vi "Lab Panel V6.00.vi"() -> ()   [LabVIEW 2017]
uses:
  sub vi/SelectLAB0X-N.ctl
  sub vi/SIG LAB0X-N.ctl
  sub vi/Set LAB0X-N.ctl
  <vilib>/Platform/TimedLoop/XDataNode/timing_clust.ctl
  <vilib>/Platform/TimedLoop/XDataNode/nitl_modes.ctl
  <vilib>/Platform/TimedLoop/XDataNode/wakeup.ctl
  Global 1.vi
  Global display 4.vi
  Global display 3.vi
  Global display 1.vi
  Global display 2.vi
  <vilib>/platform/TimedLoop/XDataNode/XDataNode.xnode
  <vilib>/Platform/TimedLoop/XDataNode/XDNodeRunTimeDep.lvlib
  sub vi/Web Imge control.ctl
panel:
  out "Loop Time":u32
  out "Process AIs":bool
  in  "path to JPEG file":path=path "C:/Users/Mike/Documents/Crabtree/Crabtree/Hardware/crabtree"
  out "Simulate IND":bool
  out "network error":bool
  out "TEMP":bool
  out "AI":bool
  out "Amb Temp":dbl format="%#.0f"
  out "Temp Up":dbl
  in  "stop all":bool
  in  "ADMIN":bool
  in  "Tab Control 2":T1(tab)
  out "SIG LAB05-2":T2 {"PF" format="%.2f"; "AMPS" format="%.1f"}
  out "SIG LAB05-1":T2 {"PF" format="%.2f"; "AMPS" format="%.1f"}
  out "SIG LAB04-2":T2 {"PF" format="%.2f"; "AMPS" format="%.1f"}
  out "SIG LAB04-1":T2 {"PF" format="%.2f"; "AMPS" format="%.1f"}
  out "SIG LAB03-2":T2 {"PF" format="%.2f"; "AMPS" format="%.1f"}
  out "SIG LAB03-1":T2 {"PF" format="%.2f"; "AMPS" format="%.1f"}
  out "SIG LAB02-2":T2 {"PF" format="%.2f"; "AMPS" format="%.1f"}
  in  "RUN LAB01-1":bool
  in  "O/I  LAB05-1":bool
  in  "O/I  LAB05-2":bool
  in  "O/I  LAB04-1":bool
  in  "O/I  LAB04-2":bool
  in  "O/I  LAB02-1":bool
  in  "O/I  LAB02-2":bool
  in  "O/I  LAB01-2":bool
  in  "O/I  LAB01-1":bool
  in  "O/I  LAB03-1":bool
  in  "RUN LAB05-2":bool
  in  "RUN LAB05-1":bool
  in  "RUN LAB04-2":bool
  in  "RUN LAB04-1":bool
  in  "RUN LAB03-2":bool
  in  "RUN LAB03-1":bool
  in  "RUN LAB02-2":bool
  in  "RUN LAB02-1":bool
  in  "RUN LAB01-2":bool
  in  "SELECT LAB05-2":T3
  in  "SELECT LAB05-1":T3
  in  "SELECT LAB04-2":T3
  in  "SELECT LAB04-1":T3
  in  "SELECT LAB03-2":T3
  in  "SELECT LAB03-1":T3
  in  "SELECT LAB02-2":T3
  in  "SELECT LAB02-1":T3
  in  "SELECT LAB01-2":T3
  in  "SELECT LAB01-1":T3
  in  "O/I  LAB03-2":bool
  out "SIG LAB01-1":T2 {"PF" format="%.2f"; "AMPS" format="%.1f"}
  out "SIG LAB01-2":T2 {"PF" format="%.2f"; "AMPS" format="%.1f"}
  out "SIG LAB02-1":T2 {"PF" format="%.2f"; "AMPS" format="%.1f"}
  out "DISP LAB05-2":T4 {"MINS" format="%.2g"}
  out "DISP LAB05-1":T4 {"MINS" format="%.2g"}
  out "DISP LAB04-2":T4 {"MINS" format="%.2g"}
  out "DISP LAB04-1":T4 {"MINS" format="%.2g"}
  out "DISP LAB03-2":T4 {"MINS" format="%.2g"}
  out "DISP LAB03-1":T4 {"MINS" format="%.2g"}
  in  "SET LAB05-2":T5={"NAME"="", "DESCRIPTION"="", "CYCLES"=5.0, "T-RISE mins"=0.0, "T-RISE deg C"=0.0} {"CYCLES" min=5.0 step=1.0}
  in  "SET LAB05-1":T5={"NAME"="", "DESCRIPTION"="", "CYCLES"=5.0, "T-RISE mins"=0.0, "T-RISE deg C"=0.0} {"CYCLES" min=5.0 step=1.0}
  in  "SET LAB04-2":T5={"NAME"="", "DESCRIPTION"="", "CYCLES"=5.0, "T-RISE mins"=0.0, "T-RISE deg C"=0.0} {"CYCLES" min=5.0 step=1.0}
  in  "SET LAB04-1":T5={"NAME"="", "DESCRIPTION"="", "CYCLES"=5.0, "T-RISE mins"=0.0, "T-RISE deg C"=0.0} {"CYCLES" min=5.0 step=1.0}
  in  "SET LAB03-2":T5={"NAME"="", "DESCRIPTION"="", "CYCLES"=5.0, "T-RISE mins"=0.0, "T-RISE deg C"=0.0} {"CYCLES" min=5.0 step=1.0}
  in  "SET LAB03-1":T5={"NAME"="", "DESCRIPTION"="", "CYCLES"=5.0, "T-RISE mins"=0.0, "T-RISE deg C"=0.0} {"CYCLES" min=5.0 step=1.0}
  out "DISP LAB02-2":T4 {"MINS" format="%.2g"}
  out "DISP LAB02-1":T4 {"MINS" format="%.2g"}
  in  "SET LAB02-2":T5={"NAME"="", "DESCRIPTION"="", "CYCLES"=5.0, "T-RISE mins"=0.0, "T-RISE deg C"=0.0} {"CYCLES" min=5.0 step=1.0}
  in  "SET LAB02-1":T5={"NAME"="", "DESCRIPTION"="", "CYCLES"=5.0, "T-RISE mins"=0.0, "T-RISE deg C"=0.0} {"CYCLES" min=5.0 step=1.0}
  out "RESULT LAB05-2":bool
  out "RESULT LAB05-1":bool
  out "RESULT LAB04-2":bool
  out "RESULT LAB04-1":bool
  out "RESULT LAB03-2":bool
  out "RESULT LAB03-1":bool
  out "RESULT LAB02-2":bool
  out "RESULT LAB02-1":bool
  out "RESULT LAB01-2":bool
  out "RESULT LAB01-1":bool
  in  "SET LAB01-1":T6={"NAME"="", "DESCRIPTION"="", "CYCLES"=5.0, "T-RISE mins"=0.0, "T-RISE deg C"=0.0} {"CYCLES" min=5.0 step=1.0}
  in  "SET LAB01-2":T5={"NAME"="", "DESCRIPTION"="", "CYCLES"=5.0, "T-RISE mins"=0.0, "T-RISE deg C"=0.0} {"CYCLES" min=5.0 step=1.0}
  out "DISP LAB01-1":T4 {"MINS" format="%.2g"}
  out "DISP LAB01-2":T4 {"MINS" format="%.2f"}
  out "TEMP RISE LAB05-2":cluster{"TL":dbl, "TN":dbl}
  out "TEMP RISE LAB05-1":cluster{"TL":dbl, "TN":dbl}
  out "TEMP RISE LAB04-2":cluster{"TL":dbl, "TN":dbl}
  out "TEMP RISE LAB04-1":cluster{"TL":dbl, "TN":dbl}
  out "TEMP RISE LAB03-2":cluster{"TL":dbl, "TN":dbl}
  out "TEMP RISE LAB03-1":cluster{"TL":dbl, "TN":dbl}
  out "TEMP RISE LAB02-2":cluster{"TL":dbl, "TN":dbl}
  out "TEMP RISE LAB02-1":cluster{"TL":dbl, "TN":dbl}
  out "TEMP RISE LAB01-2":cluster{"TL":dbl, "TN":dbl}
  out "TEMP RISE LAB01-1":cluster{"TL":dbl, "TN":dbl}
  out "JIG LAB05-2":bool
  out "JIG LAB05-1":bool
  out "JIG LAB04-2":bool
  out "JIG LAB04-1":bool
  out "JIG LAB03-2":bool
  out "JIG LAB03-1":bool
  out "JIG LAB02-2":bool
  out "JIG LAB02-1":bool
  out "JIG LAB01-2":bool
  out "JIG LAB01-1":bool
  out "TEMP START LAB01-1":cluster{"TL":dbl, "TN":dbl}
  out "TEMP START LAB02-1":cluster{"TL":dbl, "TN":dbl}
  out "TEMP START LAB03-1":cluster{"TL":dbl, "TN":dbl}
  out "TEMP START LAB04-1":cluster{"TL":dbl, "TN":dbl}
  out "TEMP START LAB01-2":cluster{"TL":dbl, "TN":dbl}
  out "TEMP START LAB02-2":cluster{"TL":dbl, "TN":dbl}
  out "TEMP START LAB03-2":cluster{"TL":dbl, "TN":dbl}
  out "TEMP START LAB04-2":cluster{"TL":dbl, "TN":dbl}
  out "TEMP START LAB05-2":cluster{"TL":dbl, "TN":dbl}
  out "TEMP START LAB05-1":cluster{"TL":dbl, "TN":dbl}
  out "LOG LAB05-2":string
  out "LOG LAB04-2":string
  out "LOG LAB03-2":string
  out "LOG LAB02-2":string
  out "LOG LAB01-2":string
  out "LOG LAB05-1":string
  out "LOG LAB04-1":string
  out "LOG LAB03-1":string
  out "LOG LAB02-1":string
  out "LOG LAB01-1":string
  in  "Tab charts":T7(tab)
  out "LAB01 VOLTS":dynamicdata(graph)
  out "LAB01 AMPS":dynamicdata(graph)
  out "LAB01 deg C":dynamicdata(graph)
  out "LAB02 VOLTS":dynamicdata(graph)
  out "LAB02 AMPS":dynamicdata(graph)
  out "LAB02 deg C":dynamicdata(graph)
  out "LAB03 VOLTS":dynamicdata(graph)
  out "LAB03 AMPS":dynamicdata(graph)
  out "LAB03 deg C":dynamicdata(graph)
  out "LAB04 VOLTS":dynamicdata(graph)
  out "LAB04 AMPS":dynamicdata(graph)
  out "LAB04 deg C":dynamicdata(graph)
  out "LAB05 VOLTS":dynamicdata(graph)
  out "LAB05 AMPS":dynamicdata(graph)
  out "LAB05 deg C":dynamicdata(graph)
  out "Reset Error":bool
  out "Er USB#2":dbl
  out "Er USB#1":dbl
  out "Er USB#0":dbl
  out "Resets Done":dbl
  out "Error USB #2":bool
  out "Error USB #1":bool
  out "Error USB #0":bool
  in  "MAIL SETTINGS":T8
  out "MAIL REPORT":string
  in  "TO (string):":string
  in  "Send Mail Now":bool
  in  "Auto Mail Send":bool
  in  "Network Directory":path
  in  "JIG ON TIME (S)":dbl=1.0 min=1.0 max=10.0 step=0.5 format="%.1g"
  in  "JIG OFF TIME (S)":dbl=2.0 min=2.0 max=10.0 step=0.5 format="%.1g"
  in  "Reset Measuring":bool
  out "path":path
  out "physical channels 0":string="DemoDevice,BID#0/ai0:1" caption="property value"
  out "physical channels 1":string="DemoDevice,BID#0/ai0:1" caption="property value"
  out "physical channels 2":string="DemoDevice,BID#0/ai0:1" caption="property value"
  in  "Min I":dbl=1.0
  in  "Min V":dbl=10.0
  out "JIG RELAY CYCLES":T9
  out "ON L05-2":cluster{"amps":dbl, "volts":dbl, "pf":dbl}
  out "ON L05-1":cluster{"amps":dbl, "volts":dbl, "pf":dbl}
  out "FAIL LAB05-2":cluster{"LO":dbl, "HI":dbl}
  out "FAIL LAB05-1":cluster{"LO":dbl, "HI":dbl}
  out "FAIL LAB04-2":cluster{"LO":dbl, "HI":dbl}
  out "FAIL LAB04-1":cluster{"LO":dbl, "HI":dbl}
  out "FAIL LAB03-2":cluster{"LO":dbl, "HI":dbl}
  out "FAIL LAB03-1":cluster{"LO":dbl, "HI":dbl}
  out "FAIL LAB02-2":cluster{"LO":dbl, "HI":dbl}
  out "FAIL LAB02-1":cluster{"LO":dbl, "HI":dbl}
  out "FAIL LAB01-2":cluster{"LO":dbl, "HI":dbl}
  out "FAIL LAB01-1":cluster{"LO":dbl, "HI":dbl}
  out "ON L01-1":cluster{"amps":dbl, "volts":dbl, "pf":dbl}
  out "ON L01-2":cluster{"amps":dbl, "volts":dbl, "pf":dbl}
  out "ON L02-1":cluster{"amps":dbl, "volts":dbl, "pf":dbl}
  out "ON L02-2":cluster{"amps":dbl, "volts":dbl, "pf":dbl}
  out "ON L03-1":cluster{"amps":dbl, "volts":dbl, "pf":dbl}
  out "ON L03-2":cluster{"amps":dbl, "volts":dbl, "pf":dbl}
  out "ON L04-1":cluster{"amps":dbl, "volts":dbl, "pf":dbl}
  out "ON L04-2":cluster{"amps":dbl, "volts":dbl, "pf":dbl}
  in  "Open Com Port":bool
  out "LA05-2 (TN)":bool
  out "LA05-2 (TL)":bool
  out "LA05-1 (TN)":bool
  out "LA05-1 (TL)":bool
  out "LA04-2 (TN)":bool
  out "LA04-2 (TL)":bool
  out "LA04-1 (TN)":bool
  out "LA04-1 (TL)":bool
  out "LA03-2 (TN)":bool
  out "LA03-2 (TL)":bool
  out "LA03-1 (TN)":bool
  out "LA03-1 (TL)":bool
  out "LA02-2 (TN)":bool
  out "LA02-2 (TL)":bool
  out "LA02-1 (TN)":bool
  out "LA02-1 (TL)":bool
  out "LA01-2 (TN)":bool
  out "LA01-2 (TL)":bool
  out "LA01-1 (TN)":bool
  out "LA01-1 (TL)":bool
  out "TEMP LA05":T10
  out "TEMP LA04":T10
  out "TEMP LA03":T10
  out "TEMP LA02":T10
  out "TEMP LA01":T10
  out "Ref deg C":dbl format="%#.0f"
  out "Temp read loop":dbl
  out "Com Port Status":bool
  out "Com setup loops":i32
  out "VISA Com out":refnum<visa-resource-name>
  in  "Select COM port":refnum<visa-resource-name>="COM6"
  in  "Read Temp":bool
  out "Error Temp":bool
  out "Fault Counters":u64[](array[numeric])
  out "TempErrors":bool[](array[boolean])
  in  "Temp Simulate":bool
  out "AI Task":bool
  out "AI Task2":u32
  out "AI Task1":u32
  out "AI Task0":u64
  out "Total USB resets":dbl
  in  "Auto Reset":bool
  in  "Mail Test File To:":string
  in  "Mail Test Fail":bool
  out "graph flag":bool
  in  "Temp Test Cal":dbl
  in  "Amps Fail level":dbl
  in  "Fail Loops":dbl
  out "Save JC":bool
  in  "DAQ Simulate":bool
  in  "Temp Value":dbl
  in  "Temp Delay Lps":dbl
  in  "SAMPLES":dbl
  in  "RATE (Hz)":dbl
  in  "JIG TEST":T11
  in  "C drive data root dir":path
  out "run lab05-2":bool
  out "run lab05-1":bool
  out "run lab04-2":bool
  out "run lab04-1":bool
  out "run lab03-2":bool
  out "run lab03-1":bool
  out "run lab02-2":bool
  out "run lab02-1":bool
  out "run lab01-2":bool
  out "run lab01-1":bool
  in  "Tab Control":T12(tab)
  out "LAB01-2 (GRAPH)":dynamicdata(graph)
  out "LAB01-1 (GRAPH)":dynamicdata(graph)
  out "LAB02-2 (GRAPH)":dynamicdata(graph)
  out "LAB02-1 (GRAPH)":dynamicdata(graph)
  out "LAB03-2 (GRAPH)":dynamicdata(graph)
  out "LAB03-1 (GRAPH)":dynamicdata(graph)
  out "LAB04-2 (GRAPH)":dynamicdata(graph)
  out "LAB04-1 (GRAPH)":dynamicdata(graph)
  out "LAB05-2 (GRAPH)":dynamicdata(graph)
  out "LAB05-1 (GRAPH)":dynamicdata(graph)
  out "Any Test Running":bool
  out "Read Time":dbl
  out "LAB05 TEMP":T13
  out "LAB04 TEMP":T13
  out "LAB02 TEMP":T13
  out "LAB01 TEMP":T13
  out "LAB03 TEMP":T13
  out "LAB05-TP":bool
  out "LAB04-TP":bool
  out "LAB03-TP":bool
  out "LAB02-TP":bool
  out "LAB01-TP":bool
  out "Analog error":bool
  out "USB OUT 0":bool[](array[boolean])
  out "USB OUT 1":bool[](array[boolean])
  out "USB OUT 2":bool[](array[boolean])
  in  "Ambient Volts":dbl format="%.2f"
  in  "PF":dbl min=0.0 max=1.0 step=0.1 format="%#.1f"
  in  "VOLTS":dbl
  in  "OFF amps":dbl min=0.0 max=100.0 step=0.1 format="%#.1f"
  in  "ON amps":dbl
  in  "LAB deg C":T14
  out "AI data 0":waveform(dbl)[](array[waveform])
  out "AI data 1":waveform(dbl)[](array[waveform])
  out "AI data 2":waveform(dbl)[](array[waveform])
  out "AI Error":errorcluster[](array[cluster])
  out "AI loop time":dbl format="%.6g"
  out "loops":dbl
  out "on loops":dbl format="%#.0f"
  out "off loops":dbl format="%#.0f"
  out "jig cycle":dbl
  out "TDMS LAB01-1":refnum<k34>
  out "data file error":errorcluster
  out "TDMS LAB02-1":refnum<k34>
  out "TDMS LAB01-2":refnum<k34>
  out "TDMS LAB02-2":refnum<k34>
  out "TDMS LAB03-1":refnum<k34>
  out "TDMS LAB03-2":refnum<k34>
  out "TDMS LAB04-1":refnum<k34>
  out "TDMS LAB04-2":refnum<k34>
  out "TDMS LAB05-1":refnum<k34>
  out "TDMS LAB05-2":refnum<k34>
  out "mail control":string
  out "File Time Stamp":timestamp
  in  "stop":bool
  out "deg C (volts)":dbl
  out "Application Directory":path
  out "ACQ Init TIme":u32
  out "ACQ Time":u32
  out "Web Server:Root Directory Path":path
  out "Analog Fault Counts":i32[](array[numeric])
  out "TEMP REF cal":dbl
  out "CAL LAB01":T15 {"2 (TN) cal" min=0.0 step=0.01 format="%.2f"; "2 (TL) cal" min=0.0 step=0.01 format="%.2f"; "2 (PF) cal" min=0.0 step=0.01 format="%.2f"; "2 (V) cal" min=0.0 step=0.01 format="%.2f"; "2 (A) cal" min=0.0 step=0.01 format="%.2f"; "1 (TN) cal" min=0.0 step=0.01 format="%.2f"; "1 (TL) cal" min=0.0 step=0.01 format="%.2f"; "1 (PF) cal" min=0.0 step=0.01 format="%.2f"; "1 (V) cal" min=0.0 step=0.01 format="%.2f"; "1  (A) cal" min=0.0 step=0.01 format="%.2f"}
  out "CAL LAB03":T15 {"2 (TN) cal" min=0.0 step=0.01 format="%.2f"; "2 (TL) cal" min=0.0 step=0.01 format="%.2f"; "2 (PF) cal" min=0.0 step=0.01 format="%.2f"; "2 (V) cal" min=0.0 step=0.01 format="%.2f"; "2 (A) cal" min=0.0 step=0.01 format="%.2f"; "1 (TN) cal" min=0.0 step=0.01 format="%.2f"; "1 (TL) cal" min=0.0 step=0.01 format="%.2f"; "1 (PF) cal" min=0.0 step=0.01 format="%.2f"; "1 (V) cal" min=0.0 step=0.01 format="%.2f"; "1  (A) cal" min=0.0 step=0.01 format="%.2f"}
  out "CAL LAB02":T16 {"2 (TN) cal" min=0.0 step=0.01 format="%.2f"; "2 (TL) cal" min=0.0 step=0.01 format="%.2f"; "2 (PF) cal" min=0.0 step=0.01 format="%.2f"; "2 (V) cal" min=0.0 step=0.01 format="%.2f"; "2 (A) cal" min=0.0 step=0.01 format="%.2f"; "1 (TN) cal" min=0.0 step=0.01 format="%.2f"; "1 (TL) cal" min=0.0 step=0.01 format="%.2f"; "1 (PF) cal" min=0.0 step=0.01 format="%.2f"; "1 (V) cal" min=0.0 step=0.01 format="%.2f"; "1 (A) cal" min=0.0 step=0.01 format="%.2f"}
  out "CAL LAB05":T15 {"2 (TN) cal" min=0.0 step=0.01 format="%.2f"; "2 (TL) cal" min=0.0 step=0.01 format="%.2f"; "2 (PF) cal" min=0.0 step=0.01 format="%.2f"; "2 (V) cal" min=0.0 step=0.01 format="%.2f"; "2 (A) cal" min=0.0 step=0.01 format="%.2f"; "1 (TN) cal" min=0.0 step=0.01 format="%.2f"; "1 (TL) cal" min=0.0 step=0.01 format="%.2f"; "1 (PF) cal" min=0.0 step=0.01 format="%.2f"; "1 (V) cal" min=0.0 step=0.01 format="%.2f"; "1  (A) cal" min=0.0 step=0.01 format="%.2f"}
  out "CAL LAB04":T15 {"2 (TN) cal" min=0.0 step=0.01 format="%.2f"; "2 (TL) cal" min=0.0 step=0.01 format="%.2f"; "2 (PF) cal" min=0.0 step=0.01 format="%.2f"; "2 (V) cal" min=0.0 step=0.01 format="%.2f"; "2 (A) cal" min=0.0 step=0.01 format="%.2f"; "1 (TN) cal" min=0.0 step=0.01 format="%.2f"; "1 (TL) cal" min=0.0 step=0.01 format="%.2f"; "1 (PF) cal" min=0.0 step=0.01 format="%.2f"; "1 (V) cal" min=0.0 step=0.01 format="%.2f"; "1  (A) cal" min=0.0 step=0.01 format="%.2f"}
  out "cal file error out":errorcluster
  in  "SET (cal)":bool
  out "AI Data 0":waveform(dbl)[](graph)
  out "AI Data 1":waveform(dbl)[](graph)
  out "AI Data 2":waveform(dbl)[](graph)
  # "v6.28"
  # "LAB01"
  # "LAB02"
  # "LAB03"
  # "LAB04"
  # "LAB05"
  # "LAB01"
  # "LAB02"
  # "LAB03"
  # "LAB04"
  # "LAB05"
  # "PANEL ID / DATE / TIME / NAME / DESCRIPTION / CYCLES / TEST TIME / STATUS"
  # "PANEL ID / DATE / TIME / NAME / DESCRIPTION / CYCLES / TEST TIME / STATUS"
  # "http://This IP:8000/Lab_Panel"
  # "(Enter recipients address seperated by comma)"
  # "JIG SET"
  # "Temperature circuits \ndetected at start up."
  # "PANEL CONTROL TO BE ON"
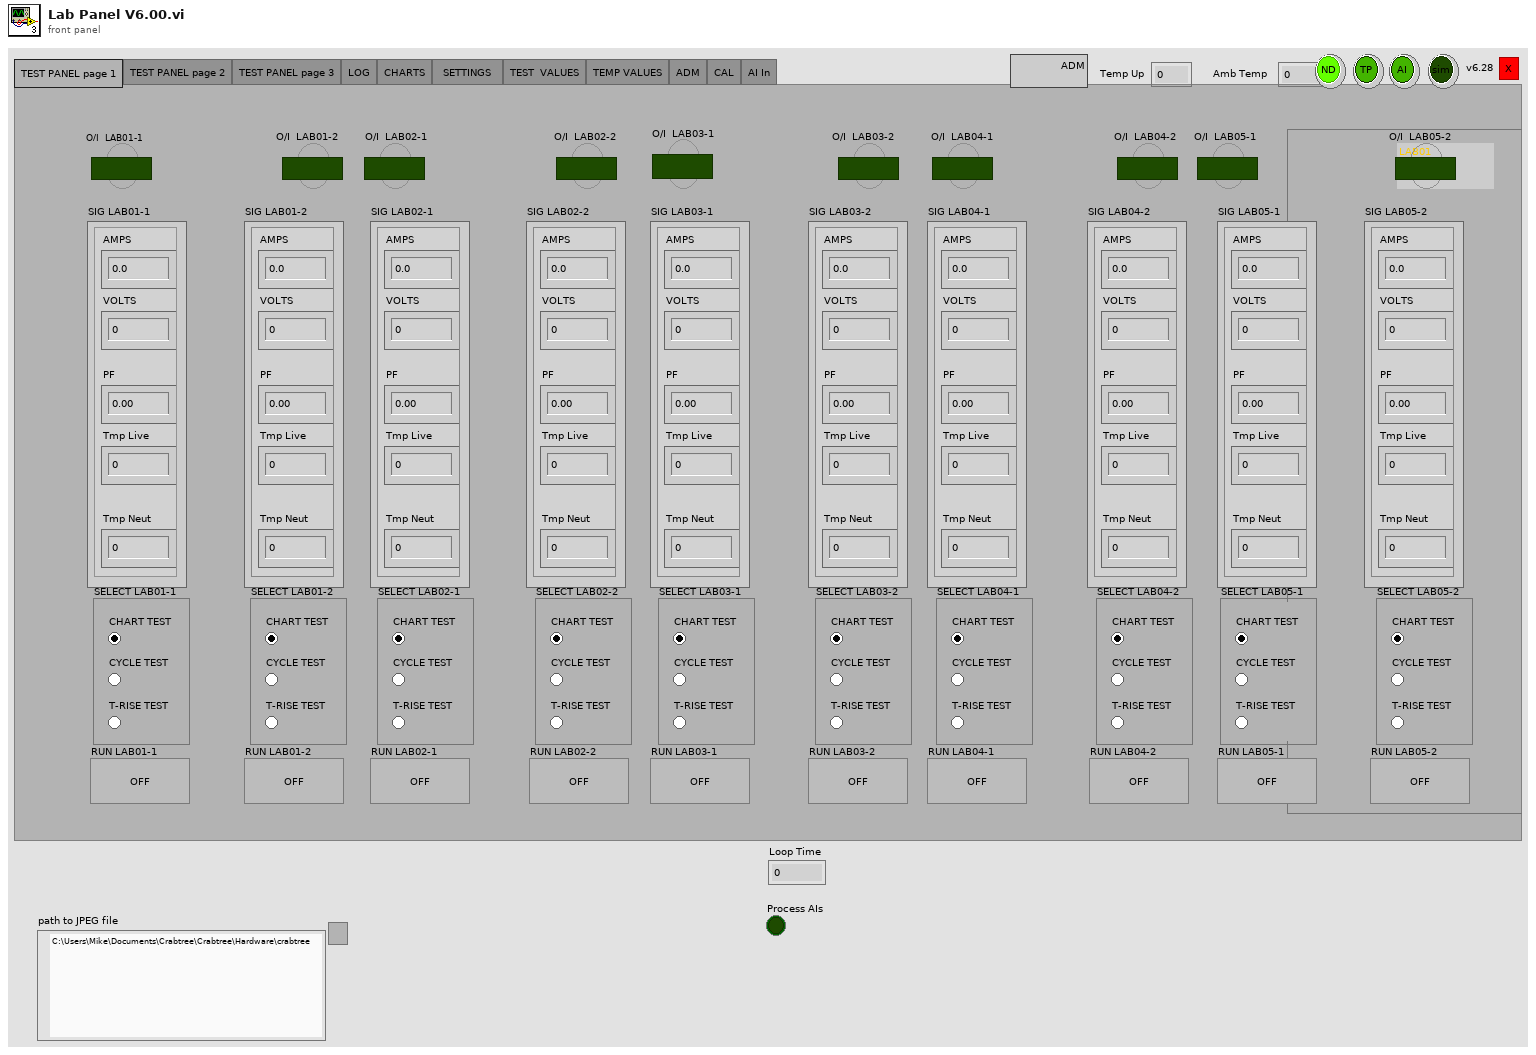
[diagram p1: front panel]
types:
  T1 = enum32{"TEST PANEL page 1", "TEST PANEL page 2", "TEST PANEL page 3", "LOG", "CHARTS", "SETTINGS   ", "TEST  VALUES", "TEMP VALUES", "ADM", "CAL", "AI In"}
  T2 = typedef "SIG LAB0X-N.ctl" = cluster{"AMPS":dbl, "VOLTS":dbl, "PF":dbl, "Tmp Live":dbl, "Tmp Neut":dbl}
  T3 = typedef "SelectLAB0X-N.ctl" = enum32{"CHART TEST", "CYCLE TEST", "T-RISE TEST"}
  T4 = cluster{"CYCLE":dbl, "MINS":dbl, "STATUS":string}
  T5 = cluster{"NAME":string, "DESCRIPTION":string, "CYCLES":dbl, "T-RISE mins":dbl, "T-RISE deg C":dbl}
  T6 = typedef "Set LAB0X-N.ctl" = cluster{"NAME":string, "DESCRIPTION":string, "CYCLES":dbl, "T-RISE mins":dbl, "T-RISE deg C":dbl}
  T7 = enum32{"LAB01", "LAB02", "LAB03", "LAB04", "LAB05"}
  T8 = cluster{"OUT SERVER ADDRESS":string, "FROM ACCOUNT":string, "USER NAME":string, "PASSWORD":string, "TEST MAIL":bool, "TEST MAIL STATUS":string, "mail error":errorcluster}
  T9 = cluster{"LAB01-1":dbl, "LAB01-2":dbl, "LAB02-1":dbl, "LAB02-2":dbl, "LAB03-1":dbl, "LAB03-2":dbl, "LAB04-1":dbl, "LAB04-2":dbl, "LAB05-1":dbl, "LAB05-2":dbl}
  T10 = cluster{"TL-1":dbl, "TN-1":dbl, "TL-2":dbl, "TN-2":dbl, "TL -1COUNT":dbl, "TN-1 COUNT":dbl, "TL-2 COUNT":dbl, "TN-2 COUNT":dbl}
  T11 = cluster{" LAB01-1":bool, " LAB01-2":bool, "LAB02-1":bool, " LAB02-2":bool, "LAB03-1":bool, "LAB03-2":bool, "LAB04-1":bool, "LAB04-2":bool, "LAB05-1":bool, "LAB05-2":bool}
  T12 = enum32{"LAB01", "LAB02", "LAB03", "LAB04", "LAB05", "TEMPERATURE", "GENERAL INFO", "Simulate", "AI Data Out"}
  T13 = cluster{"T1 Live":dbl, "T1 Neut":dbl, "T2 Live":dbl, "T2 Neut":dbl, "ID":dbl, "ER":dbl}
  T14 = cluster{"1 TL":dbl, "1 TN":dbl, "2 TL":dbl, "2 TN":dbl, "ID":dbl, "ER":dbl}
  T15 = cluster{"1  (A) cal":dbl, "1 (V) cal":dbl, "1 (PF) cal":dbl, "1 (TL) cal":dbl, "1 (TN) cal":dbl, "2 (A) cal":dbl, "2 (V) cal":dbl, "2 (PF) cal":dbl, "2 (TL) cal":dbl, "2 (TN) cal":dbl}
  T16 = cluster{"1 (A) cal":dbl, "1 (V) cal":dbl, "1 (PF) cal":dbl, "1 (TL) cal":dbl, "1 (TN) cal":dbl, "2 (A) cal":dbl, "2 (V) cal":dbl, "2 (PF) cal":dbl, "2 (TL) cal":dbl, "2 (TN) cal":dbl}
  T17 = enum8{"Enabled", "Disabled", "Disabled and Grayed Out"}
  T18 = enum16{"open", "replace", "create", "open or create", "replace or create", "replace or create with confirmation"}
  T19 = typedef "XDNodeRunTimeDep.lvlib/timing_clust.ctl" = cluster{"Expected End [f-1]":u64, "Actual End [f-1]":u64, "Finished Late? [f-1]":bool, "Expected End [i-1]":u64, "Actual End [i-1]":u64, "Finished Late? [i-1]":bool, "Expected Start [i]":u64, "Actual Start [i]":u64, "Expected Start [f]":u64, "Actual Start [f]":u64, "Source Name":string, "Structure Name":string, "Period":i64, "Deadline":i64, "Offset":i64, "Start":i64, "Priority":i32, "Timeout":i32, "Mode":T20, "Wakeup Reason":T21, "Error":errorcluster, "Source Type":string, "Secondary Source Type":string, "Global End Time":u64, "Global Start Time":u64, "Frame Duration":u64, "Iteration Duration":u64, "Assigned CPU":i32, "I/O Scan Engine Mode":u32}
  T20 = typedef "XDNodeRunTimeDep.lvlib/nitl_modes.ctl" = enum32{"No Change", "Process missed periods, maintain original phase", "Discard missed periods, maintain original phase", "Process missed periods, ignore original phase", "Discard missed periods, ignore original phase"}
  T21 = typedef "XDNodeRunTimeDep.lvlib/wakeup.ctl" = enum32{"Normal", "Aborted", "Asynchronous wakeup", "Timing source error", "Timed loop error", "Timeout"}
  T22 = enum16{"open", "open or create", "create or replace", "create", "open (read-only)"}
  T23 = cluster{"status":string, "mail server":string, "mail from":string, "mail to":string, "mail file":bool}
  T24 = typedef "Web Imge control.ctl" = cluster{"Tab Ref":refnum<vi>, "Values":i32[]}
  T25 = cluster{"SET LAB01-1":T6, "SET LAB01-2":cluster{"NAME":string, "DESCRIPTION":string, "CYCLES":dbl, "T-RISE mins":dbl, "T-RISE deg C":dbl}, "SET LAB02-1":cluster{"NAME":string, "DESCRIPTION":string, "CYCLES":dbl, "T-RISE mins":dbl, "T-RISE deg C":dbl}, "SET LAB02-2":cluster{"NAME":string, "DESCRIPTION":string, "CYCLES":dbl, "T-RISE mins":dbl, "T-RISE deg C":dbl}, "SET LAB03-1":cluster{"NAME":string, "DESCRIPTION":string, "CYCLES":dbl, "T-RISE mins":dbl, "T-RISE deg C":dbl}, "SET LAB03-2":cluster{"NAME":string, "DESCRIPTION":string, "CYCLES":dbl, "T-RISE mins":dbl, "T-RISE deg C":dbl}, "SET LAB04-1":cluster{"NAME":string, "DESCRIPTION":string, "CYCLES":dbl, "T-RISE mins":dbl, "T-RISE deg C":dbl}, "SET LAB04-2":cluster{"NAME":string, "DESCRIPTION":string, "CYCLES":dbl, "T-RISE mins":dbl, "T-RISE deg C":dbl}, "SET LAB05-1":cluster{"NAME":string, "DESCRIPTION":string, "CYCLES":dbl, "T-RISE mins":dbl, "T-RISE deg C":dbl}, "SET LAB05-2":cluster{"NAME":string, "DESCRIPTION":string, "CYCLES":dbl, "T-RISE mins":dbl, "T-RISE deg C":dbl}, "Network Directory":path, "C drive data root dir":path, "RATE (Hz)":dbl, "SAMPLES":dbl, "Select COM port":refnum<visa-resource-name>, "Temp Delay Lps":dbl, "Temp Value":dbl, "Fail Loops":dbl, "Temp Test Cal":dbl, "Amps Fail level":dbl, "Mail Test File To:":string, "Mail Test Fail":bool}
  T26 = cluster{"MAIL SETTINGS":cluster{"OUT SERVER ADDRESS":string, "FROM ACCOUNT":string, "USER NAME":string, "PASSWORD":string, "TEST MAIL":bool, "TEST MAIL STATUS":string, "mail error":errorcluster}, "Auto Mail Send":bool, string}
  T27 = cluster{"id1":bool, "id2":bool, "id3":bool, "id4":bool, "id5":bool}
  T28 = cluster{"T1":dbl, "T2":dbl, "T3":dbl, "T4":dbl, "ID":dbl, "ER":dbl}
  T29 = typedef "imagedata.ctl" = cluster{"image type":i32, "image depth":i32, "image":u8[], "mask":u8[], "colors":u32[], "Rectangle":cluster{"left":i16, "top":i16, "right":i16, "bottom":i16}}
  T30 = cluster{"STATUS":string, "OUT SERVER ADDRESS":string, "FROM ACCOUNT":string, "Mail Test File To:":string, "Mail Test Fail":bool}
  T31 = cluster{"LAB01-1 (A)":dbl, "LAB01-1 (V)":dbl, "LAB01-1 (PF)":dbl, "LAB01-2 (A)":dbl, "LAB01-2 (V)":dbl, "LAB01-2 (PF)":dbl}
  T32 = cluster{"LAB02-1 (A)":dbl, "LAB02-1 (V)":dbl, "LAB02-1 (PF)":dbl, "LAB02-2 (A)":dbl, "LAB02-2 (V)":dbl, "LAB02-2 (PF)":dbl}
  T33 = cluster{"LAB03-1 (A)":dbl, "LAB03-1 (V)":dbl, "LAB03-1 (PF)":dbl, "LAB03-2 (A)":dbl, "LAB03-2 (V)":dbl, "LAB03-2 (PF)":dbl}
  T34 = cluster{"LAB04-1 (A)":dbl, "LAB04-1 (V)":dbl, "LAB04-1 (PF)":dbl, "LAB04-2 (A)":dbl, "LAB04-2 (V)":dbl, "LAB04-2 (PF)":dbl}
  T35 = cluster{"LAB05-1 (A)":dbl, "LAB05-1 (V)":dbl, "LAB05-1 (PF)":dbl, "LAB05-2 (A)":dbl, "LAB05-2 (V)":dbl, "LAB05-2 (PF)":dbl}
  T36 = cluster{"OFF amps":dbl, "VOLTS":dbl, "PF":dbl, "OFF amps":dbl, "VOLTS":dbl, "PF":dbl}
  T37 = cluster{"FAIL LAB01-1":cluster{"LO":dbl, "HI":dbl}, "SIG LAB01-1":T2, "TEMP START LAB01-1":cluster{"TL":dbl, "TN":dbl}, "DISP LAB01-1":cluster{"CYCLE":dbl, "MINS":dbl, "STATUS":string}, "SET LAB01-1":T6, "TDMS LAB01-1":refnum<k34>}
  T38 = cluster{"FAIL LAB01-2":cluster{"LO":dbl, "HI":dbl}, "SIG LAB01-2":T2, "TEMP START LAB01-2":cluster{"TL":dbl, "TN":dbl}, "DISP LAB01-2":cluster{"CYCLE":dbl, "MINS":dbl, "STATUS":string}, "SET LAB01-2":cluster{"NAME":string, "DESCRIPTION":string, "CYCLES":dbl, "T-RISE mins":dbl, "T-RISE deg C":dbl}, "TDMS LAB01-2":refnum<k34>}
  T39 = cluster{"FAIL LAB02-1":cluster{"LO":dbl, "HI":dbl}, "SIG LAB02-1":T2, "TEMP START LAB02-1":cluster{"TL":dbl, "TN":dbl}, "DISP LAB02-1":cluster{"CYCLE":dbl, "MINS":dbl, "STATUS":string}, "SET LAB02-1":cluster{"NAME":string, "DESCRIPTION":string, "CYCLES":dbl, "T-RISE mins":dbl, "T-RISE deg C":dbl}, "TDMS LAB02-1":refnum<k34>}
  T40 = cluster{"FAIL LAB02-2":cluster{"LO":dbl, "HI":dbl}, "SIG LAB02-2":T2, "TEMP START LAB02-2":cluster{"TL":dbl, "TN":dbl}, "DISP LAB02-2":cluster{"CYCLE":dbl, "MINS":dbl, "STATUS":string}, "SET LAB02-2":cluster{"NAME":string, "DESCRIPTION":string, "CYCLES":dbl, "T-RISE mins":dbl, "T-RISE deg C":dbl}, "TDMS LAB02-2":refnum<k34>}
  T41 = cluster{"FAIL LAB03-1":cluster{"LO":dbl, "HI":dbl}, "SIG LAB03-1":T2, "TEMP START LAB03-1":cluster{"TL":dbl, "TN":dbl}, "DISP LAB03-1":cluster{"CYCLE":dbl, "MINS":dbl, "STATUS":string}, "SET LAB03-1":cluster{"NAME":string, "DESCRIPTION":string, "CYCLES":dbl, "T-RISE mins":dbl, "T-RISE deg C":dbl}, "TDMS LAB03-1":refnum<k34>}
  T42 = cluster{"FAIL LAB03-2":cluster{"LO":dbl, "HI":dbl}, "SIG LAB03-2":T2, "TEMP START LAB03-2":cluster{"TL":dbl, "TN":dbl}, "DISP LAB03-2":cluster{"CYCLE":dbl, "MINS":dbl, "STATUS":string}, "SET LAB03-2":cluster{"NAME":string, "DESCRIPTION":string, "CYCLES":dbl, "T-RISE mins":dbl, "T-RISE deg C":dbl}, "TDMS LAB03-2":refnum<k34>}
  T43 = cluster{"FAIL LAB04-1":cluster{"LO":dbl, "HI":dbl}, "SIG LAB04-1":T2, "TEMP START LAB04-1":cluster{"TL":dbl, "TN":dbl}, "DISP LAB04-1":cluster{"CYCLE":dbl, "MINS":dbl, "STATUS":string}, "SET LAB04-1":cluster{"NAME":string, "DESCRIPTION":string, "CYCLES":dbl, "T-RISE mins":dbl, "T-RISE deg C":dbl}, "TDMS LAB04-1":refnum<k34>}
  T44 = cluster{"FAIL LAB04-2":cluster{"LO":dbl, "HI":dbl}, "SIG LAB04-2":T2, "TEMP START LAB04-2":cluster{"TL":dbl, "TN":dbl}, "DISP LAB04-2":cluster{"CYCLE":dbl, "MINS":dbl, "STATUS":string}, "SET LAB04-2":cluster{"NAME":string, "DESCRIPTION":string, "CYCLES":dbl, "T-RISE mins":dbl, "T-RISE deg C":dbl}, "TDMS LAB04-2":refnum<k34>}
  T45 = cluster{"FAIL LAB05-1":cluster{"LO":dbl, "HI":dbl}, "SIG LAB05-1":T2, "TEMP START LAB05-1":cluster{"TL":dbl, "TN":dbl}, "DISP LAB05-1":cluster{"CYCLE":dbl, "MINS":dbl, "STATUS":string}, "SET LAB05-1":cluster{"NAME":string, "DESCRIPTION":string, "CYCLES":dbl, "T-RISE mins":dbl, "T-RISE deg C":dbl}, "TDMS LAB05-1":refnum<k34>}
  T46 = cluster{"FAIL LAB05-2":cluster{"LO":dbl, "HI":dbl}, "SIG LAB05-2":T2, "TEMP START LAB05-2":cluster{"TL":dbl, "TN":dbl}, "DISP LAB05-2":cluster{"CYCLE":dbl, "MINS":dbl, "STATUS":string}, "SET LAB05-2":cluster{"NAME":string, "DESCRIPTION":string, "CYCLES":dbl, "T-RISE mins":dbl, "T-RISE deg C":dbl}, "TDMS LAB05-2":refnum<k34>}
  T47 = cluster{"MAIL SETTINGS":cluster{"OUT SERVER ADDRESS":string, "FROM ACCOUNT":string, "USER NAME":string, "PASSWORD":string, "TEST MAIL":bool, "TEST MAIL STATUS":string, "mail error":errorcluster}, "Auto Mail Send":bool, "TO (string):":string}
  T48 = cluster{"TP1-L":dbl, "TP1-N":dbl, "TP2-L":dbl, "TP2-N":dbl, "TP1-L COUNT":dbl, "TP1-N COUNT":dbl, "TP2-L COUNT":dbl, "TP2-N COUNT":dbl}
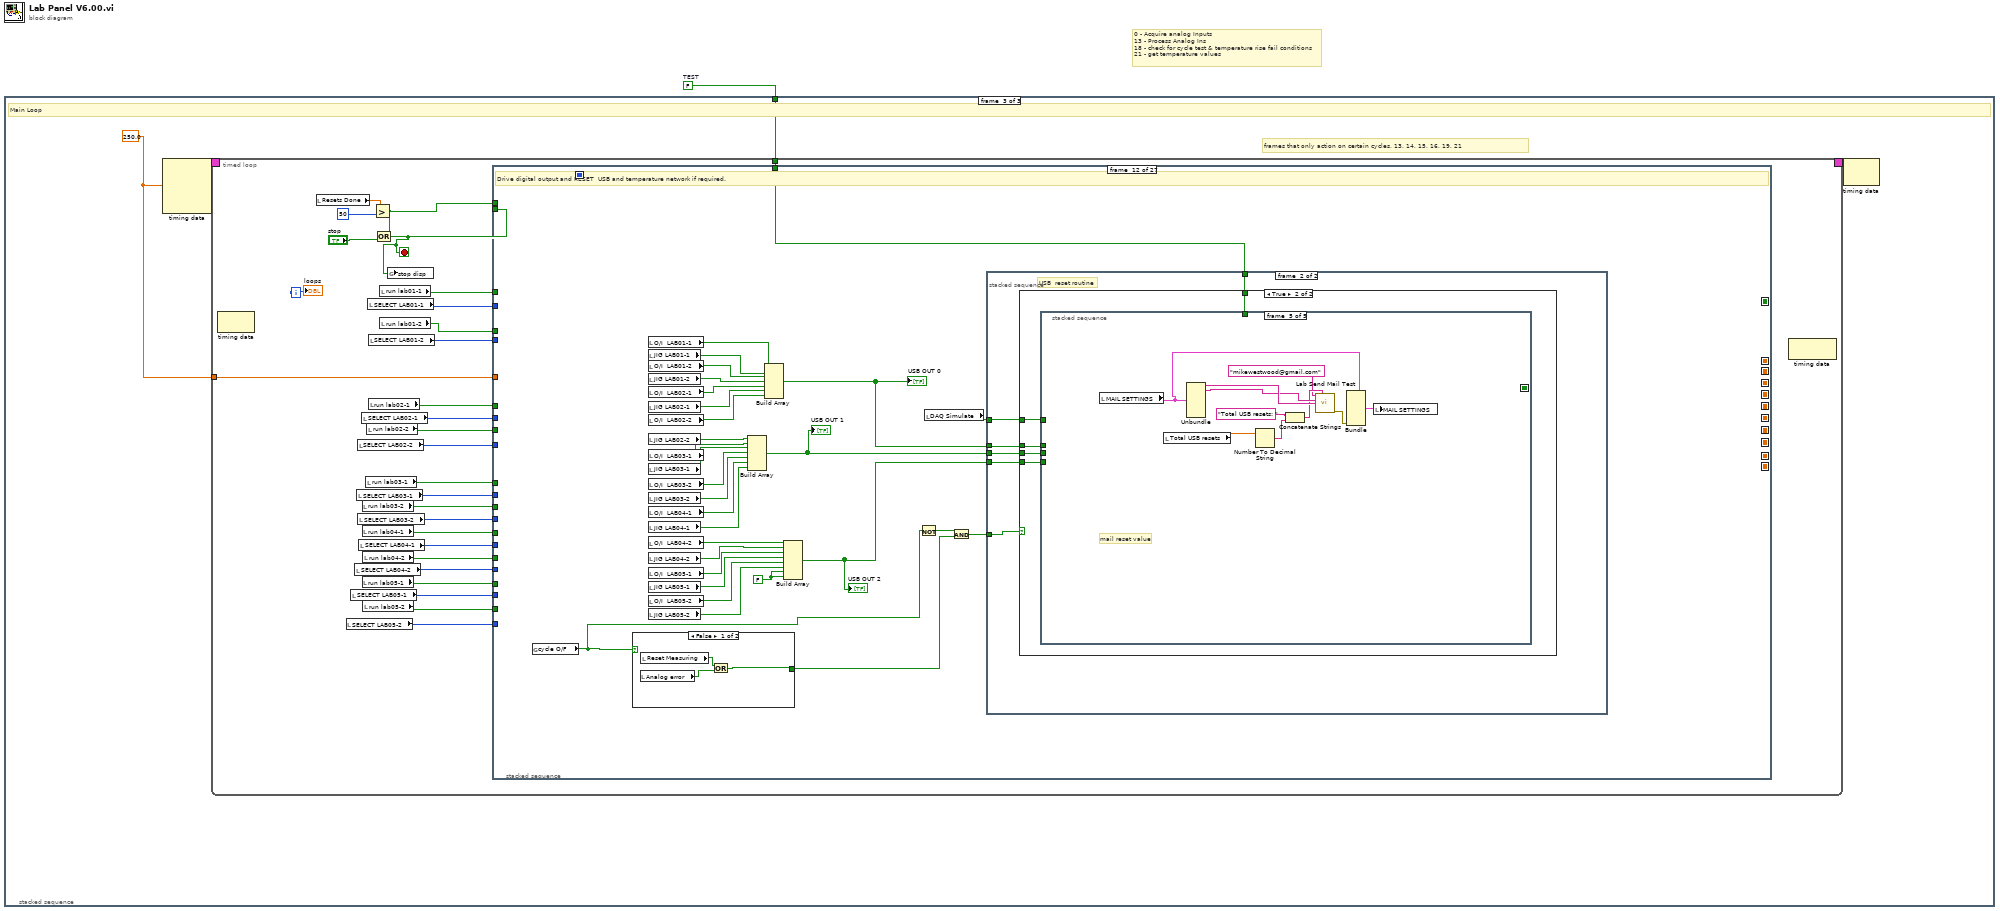
[diagram p0: block diagram]
diagram:
  w1 = FALSE  # TEST
  # "0 - Acquire analog Inputs\n13 - Process Analog Ins\n18 - check for cycle test & temperature rise fail conditions\n21 - get temperature values"
  n1 = stacked-sequence {
    tunnel: w1 -> [_ w11 w348]
    frame #0 {
      # "Front panel Terminals (???)"
      n2 = local write "Save JC"(FALSE) -> ()
      n3 = call "App Data Files and folders.vi"("ApplicationName"="Crabtree LabPanel" ("name or relative path")) -> ("Exec Log Path"=w2:path)  [unwired: 8 in, 2 out]
      n4 = call "ExecLog_CreateLog.vi"("file path"=w2) -> ()  [unwired: 5 in, 3 out]
      n5 = disable-structure shown="Disabled" {
        frame Disabled {
          n6 = Open Application Reference() -> (3:w10:refnum<vi>)  [unwired: 4 in, 1 out]
          n7 = property class="App"(reference=w10, "WebSrvr.Active"=TRUE ("Web Server:Server Active")) -> (reference out=w9:refnum<vi>, error out=w6:errorcluster, "WebSrvr.RootPath"=→"Web Server:Root Directory Path":path)  [unwired: 1 in]
          n8 = Close Reference(reference=w9) -> ()  [unwired: 1 in, 1 out]
          n9 = call <vilib>:"Simple Error Handler.vi"("error in (no error)"=w6) -> ()  [unwired: 4 in, 5 out]
        }
        frame Enabled {
        }
      }
      "jig cycle" <- 0
    }
    frame #1 {
      # "do 1st time set up"
      n10 = stacked-sequence {
        tunnel: w11 -> [_ w14 _ _ _ _ _ _ _ _ _ w332 _ _]
        frame #0 {
          # "check for simulate mode"
          n11 = call "subvi-simulate v1.vi"() -> ("Sim"=w12:bool)  [unwired: 11 in]
          n12 = case shown="True" w12 {
            frame False {
            }
            frame True {
              w13 = TRUE
              n13 = local write "Temp Simulate"(w13) -> ()
              n14 = local write "DAQ Simulate"(w13) -> ()
            }
          }
        }
        frame #1 {
          # "RESET USB AND TEMPERATURE CIRCUITS"
          n15 = local read "DAQ Simulate"() -> (w15:bool)
          n16 = case shown="False" w15 {
            tunnel: w14 -> [w16 _]
            frame False {
              n17 = call "Reset USB&temp v 1.vi"("Test"=w16) -> ()  [unwired: 10 in, 1 out]
            }
            frame True {
            }
          }
        }
        frame #2 {
          # "Disable front panel while 1st time set up is being done         -                Configure Web Server"
          n18 = disable-structure shown="Enabled" {
            frame Enabled {
              n19 = property on="Tab Control 2" class="TabCtl (strict)"() -> ("Pages"=w34:refnum<vi>[])  [unwired: 2 in, 2 out]
              n20 = Index Array(array=w34, index=8) -> (element=w32:refnum<vi>)
              n21 = property class="Page"(reference=w32, "PageVis"=FALSE) -> ()  [unwired: 1 in, 2 out]
            }
            frame Disabled {
            }
          }
          n22 = property on="Tab Control 2" class="TabCtl (strict)"("Value"=0) -> ()  [unwired: 2 in, 2 out]
          n23 = local write "ADMIN"(FALSE) -> ()
          n24 = property on="Tab Control 2" class="TabCtl (strict)"("DisabledEnum"=T17."Disabled and Grayed Out" ("Disabled")) -> ()  [unwired: 2 in, 2 out]
          n25 = call <vilib>:"Application Directory.vi"() -> ("Application Directory"=w17:path)
          n26 = Call Chain() -> (call chain=w20:string[])
          n27 = Current VI's Path() -> (path=→"path":path)
          n28 = Array Size(array=w20) -> (size(s)=w22:i32)
          n29 = Open Application Reference() -> (3:w27:refnum<vi>)  [unwired: 4 in, 1 out]
          n30 = Decrement(x=w22) -> (x-1=w21:i32)
          n31 = Index Array(array=w20, index=w21) -> (element=w19:string)
          n32 = Build Path(base path=w17, name or relative path=w19) -> (appended path=→"Application Directory":path)
          n33 = property class="App"(reference=w27, "WebSrvr.Active"=TRUE ("Web Server:Server Active"), "WebSrvr.RootPath"=w17) -> (reference out=w25:refnum<vi>, error out=w23:errorcluster)  [unwired: 1 in]
          n34 = Close Reference(reference=w25) -> ()  [unwired: 1 in, 1 out]
          n35 = call <vilib>:"Simple Error Handler.vi"("error in (no error)"=w23) -> ()  [unwired: 4 in, 5 out]
        }
        frame #3 {
          # "Get calibration values"
          n36 = call "sub vi - get calibration values v1.vi"() -> ("TEMP REF CAL"=w35:dbl, "LAB01 (CAL)"=→"CAL LAB01":T15, "LAB02 (CAL)"=→"CAL LAB02":T16, "LAB03 (CAL)"=→"CAL LAB03":T15, "LAB04 (CAL)"=→"CAL LAB04":T15, "calibration file error out"=→"cal file error out":errorcluster, "LAB05 (CAL)"=→"CAL LAB05":T15)  [unwired: 9 in]
          n37 = local write "TEMP REF cal"(w35) -> ()
        }
        frame #4 {
          # "get last saved test settings from file"
          n38 = local read "Network Directory"() -> (w64:path)
          n39 = local read "C drive data root dir"() -> (w62:path)
          n40 = local read "SET LAB05-2"() -> (w94:T5)
          n41 = local read "SAMPLES"() -> (w60:dbl)
          n42 = local read "SET LAB05-1"() -> (w95:T5)
          n43 = local read "RATE (Hz)"() -> (w61:dbl)
          n44 = local read "SET LAB04-2"() -> (w96:T5)
          n45 = local read "SET LAB03-2"() -> (w93:T5)
          n46 = local read "SET LAB04-1"() -> (w97:T5)
          n47 = local read "SET LAB03-1"() -> (w92:T5)
          n48 = local read "SET LAB02-2"() -> (w91:T5)
          n49 = local read "SET LAB02-1"() -> (w90:T5)
          n50 = local read "SET LAB01-2"() -> (w89:T5)
          n51 = local read "SET LAB01-1"() -> (w88:T6)
          n52 = local read "Select COM port"() -> (w57:refnum<visa-resource-name>)
          n53 = local read "Temp Delay Lps"() -> (w56:dbl)
          n54 = local read "Mail Test File To:"() -> (w46:string)
          n55 = local read "Temp Value"() -> (w55:dbl)
          n56 = local read "Temp Test Cal"() -> (w50:dbl)
          n57 = local read "Amps Fail level"() -> (w49:dbl)
          n58 = local read "Fail Loops"() -> (w52:dbl)
          n59 = local read "Mail Test Fail"() -> (w44:bool)
          n60 = Bundle("SET LAB01-1"=w88, "SET LAB01-2"=w89, "SET LAB02-1"=w90, "SET LAB02-2"=w91, "SET LAB03-1"=w92, "SET LAB03-2"=w93, "SET LAB04-1"=w97, "SET LAB04-2"=w96, "SET LAB05-1"=w95, "SET LAB05-2"=w94, "Network Directory"=w64, "C drive data root dir"=w62, "RATE (Hz)"=w61, "SAMPLES"=w60, "Select COM port"=w57, "Temp Delay Lps"=w56, "Temp Value"=w55, "Fail Loops"=w52, "Temp Test Cal"=w50, "Amps Fail level"=w49, "Mail Test File To:"=w46, "Mail Test Fail"=w44) -> (w81:T25)  [unwired: 1 in]
          n61 = String To Path(string="c:\\crabtree\\Set Up\\") -> (path=w85:path)
          n62 = Build Path(base path=w85, name or relative path="settings.bin") -> (appended path=w83:path)
          n63 = Create Folder(path (use dialog)=w85) -> (error out=w87:errorcluster)  [unwired: 2 in, 2 out]
          n64 = call <vilib>:"Clear Errors.vi"("error in (no error)"=w87) -> ()  [unwired: 5 in, 2 out]
          n65 = Open/Create/Replace File(file path (use dialog)=w83) -> (refnum out=w80:refnum<file>, error out=w82:errorcluster)  [unwired: 5 in, 1 out]
          n66 = Read from Binary File(5:w81, 8:w82, 11:w80) -> (0:w77:errorcluster, 2:w79:T25, 3:w78:refnum<file>)  [unwired: 3 in, 1 out]
          n67 = Unbundle(w79) -> ("SET LAB01-1"=w75:T6, "SET LAB01-2"=w74:T5, "SET LAB02-1"=w73:T5, "SET LAB02-2"=w72:T5, "SET LAB03-1"=w71:T5, "SET LAB03-2"=w70:T5, "SET LAB04-1"=w69:T5, "SET LAB04-2"=w68:T5, "SET LAB05-1"=w67:T5, "SET LAB05-2"=w66:T5, "Network Directory"=w65:path, "C drive data root dir"=w63:path, "RATE (Hz)"=w58:dbl, "SAMPLES"=w59:dbl, "Select COM port"=w42:refnum<visa-resource-name>, "Temp Delay Lps"=w54:dbl, "Temp Value"=w53:dbl, "Fail Loops"=w51:dbl, "Temp Test Cal"=w48:dbl, "Amps Fail level"=w47:dbl, "Mail Test File To:"=w45:string, "Mail Test Fail"=w43:bool)
          n68 = Close File(refnum=w78, error in=w77) -> (error out=w76:errorcluster)  [unwired: 1 out]
          n69 = local write "data file error"(w76) -> ()
          n70 = local write "Temp Test Cal"(w48) -> ()
          n71 = local write "Amps Fail level"(w47) -> ()
          n72 = local write "Mail Test File To:"(w45) -> ()
          n73 = local write "Mail Test Fail"(w43) -> ()
          n74 = local write "Fail Loops"(w51) -> ()
          n75 = local write "Temp Delay Lps"(w54) -> ()
          n76 = local write "C drive data root dir"(w63) -> ()
          n77 = local write "Temp Value"(w53) -> ()
          n78 = local write "Network Directory"(w65) -> ()
          n79 = local write "SAMPLES"(w59) -> ()
          n80 = local write "RATE (Hz)"(w58) -> ()
          n81 = local write "SET LAB04-2"(w68) -> ()
          n82 = local write "SET LAB05-1"(w67) -> ()
          n83 = local write "SET LAB04-1"(w69) -> ()
          n84 = local write "SET LAB05-2"(w66) -> ()
          n85 = local write "SET LAB02-1"(w73) -> ()
          n86 = local write "SET LAB02-2"(w72) -> ()
          n87 = local write "SET LAB03-1"(w71) -> ()
          n88 = local write "SET LAB03-2"(w70) -> ()
          n89 = local write "SET LAB01-1"(w75) -> ()
          n90 = local write "SET LAB01-2"(w74) -> ()
          n91 = local write "Select COM port"(w42) -> ()
          n92 = global write "Global 1.vi" "COM port"(w42) -> ()
        }
        frame #5 {
          # "Get total resets value from file"
          n93 = String To Path(string="c:\\crabtree\\Set Up\\") -> (path=w108:path)
          n94 = Build Path(base path=w108, name or relative path="USB resets.bin") -> (appended path=w101:path)
          n95 = Create Folder(path (use dialog)=w108) -> (error out=w100:errorcluster)  [unwired: 2 in, 2 out]
          n96 = call <vilib>:"Clear Errors.vi"("error in (no error)"=w100) -> ()  [unwired: 5 in, 2 out]
          n97 = Open/Create/Replace File(file path (use dialog)=w101, operation (0:open)=T18."open or create") -> (refnum out=w106:refnum<file>, error out=w105:errorcluster)  [unwired: 4 in, 1 out]
          n98 = local read "Total USB resets"() -> (w99:dbl)
          n99 = Read from Binary File(5:w99, 8:w105, 11:w106) -> (0:w103:errorcluster, 2:w98:dbl, 3:w104:refnum<file>)  [unwired: 3 in, 1 out]
          n100 = local write "Total USB resets"(w98) -> ()
          n101 = Close File(refnum=w104, error in=w103) -> (error out=w102:errorcluster)  [unwired: 1 out]
          n102 = local write "data file error"(w102) -> ()
        }
        frame #6 {
          # "Get last saved jig cycles value from file"
          n103 = String To Path(string="c:\\crabtree\\Jig Cycles\\") -> (path=w120:path)
          n104 = Build Path(base path=w120, name or relative path="jigcycles.bin") -> (appended path=w118:path)
          n105 = Create Folder(path (use dialog)=w120) -> (error out=w122:errorcluster)  [unwired: 2 in, 2 out]
          n106 = call <vilib>:"Clear Errors.vi"("error in (no error)"=w122) -> ()  [unwired: 5 in, 2 out]
          n107 = Open/Create/Replace File(file path (use dialog)=w118) -> (refnum out=w116:refnum<file>, error out=w117:errorcluster)  [unwired: 5 in, 1 out]
          n108 = Read from Binary File(5:T9 {"LAB01-1"=0.0, "LAB01-2"=0.0, "LAB02-1"=0.0, "LAB02-2"=0.0, "LAB03-1"=0.0, "LAB03-2"=0.0, "LAB04-1"=0.0, "LAB04-2"=0.0, "LAB05-1"=0.0, "LAB05-2"=0.0} ("JIG RELAY CYCLES"), 8:w117, 11:w116) -> (0:w114:errorcluster, 2:w111:T9, 3:w115:refnum<file>)  [unwired: 3 in, 1 out]
          n109 = local write "JIG RELAY CYCLES"(w111) -> ()
          n110 = Close File(refnum=w115, error in=w114) -> (error out=w113:errorcluster)  [unwired: 1 out]
          n111 = local write "data file error"(w113) -> ()
        }
        frame #7 {
          # "Get mail settings"
          n112 = local read "Auto Mail Send"() -> (w126:bool)
          n113 = local read "MAIL SETTINGS"() -> (w130:T8)
          n114 = String To Path(string="c:\\crabtree\\Set Up\\") -> (path=w138:path)
          n115 = Build Path(base path=w138, name or relative path="mail.bin") -> (appended path=w136:path)
          n116 = Create Folder(path (use dialog)=w138) -> (error out=w140:errorcluster)  [unwired: 2 in, 2 out]
          n117 = Bundle("MAIL SETTINGS"=w130, "Auto Mail Send"=w126, "") -> (w129:T26)  [unwired: 1 in]
          n118 = call <vilib>:"Clear Errors.vi"("error in (no error)"=w140) -> ()  [unwired: 5 in, 2 out]
          n119 = Open/Create/Replace File(file path (use dialog)=w136) -> (refnum out=w134:refnum<file>, error out=w135:errorcluster)  [unwired: 5 in, 1 out]
          n120 = Read from Binary File(5:w129, 8:w135, 11:w134) -> (0:w132:errorcluster, 2:w128:T26, 3:w133:refnum<file>)  [unwired: 3 in, 1 out]
          n121 = Close File(refnum=w133, error in=w132) -> (error out=w131:errorcluster)  [unwired: 1 out]
          n122 = local write "data file error"(w131) -> ()
          n123 = Unbundle(w128) -> ("MAIL SETTINGS"=w127:T8, "Auto Mail Send"=w125:bool, w124:string)
          n124 = local write "Auto Mail Send"(w125) -> ()
          n125 = local write "TO (string):"(w124) -> ()
          n126 = local write "MAIL SETTINGS"(w127) -> ()
        }
        frame #8 {
          # "Set display status if blank"
          n127 = local read "DISP LAB03-2"() -> (w170:T4)
          n128 = local read "DISP LAB03-1"() -> (w177:T4)
          n129 = local read "DISP LAB02-2"() -> (w184:T4)
          n130 = local read "DISP LAB01-2"() -> (w197:T4)
          n131 = local read "DISP LAB01-1"() -> (w206:T4)
          n132 = local read "DISP LAB02-1"() -> (w191:T4)
          n133 = Unbundle(w170) -> ("STATUS"=w172:string)  [unwired: 2 out]
          n134 = Unbundle(w177) -> ("STATUS"=w179:string)  [unwired: 2 out]
          n135 = Unbundle(w184) -> ("STATUS"=w186:string)  [unwired: 2 out]
          n136 = Unbundle(w191) -> ("STATUS"=w193:string)  [unwired: 2 out]
          n137 = Unbundle(w197) -> ("STATUS"=w200:string)  [unwired: 2 out]
          n138 = Unbundle(w206) -> ("STATUS"=w207:string)  [unwired: 2 out]
          n139 = Equal?(x="", y=w172) -> (x = y?=w174:bool)
          n140 = Equal?(x="", y=w179) -> (x = y?=w181:bool)
          n141 = Equal?(x="", y=w186) -> (x = y?=w188:bool)
          n142 = Equal?(x="", y=w193) -> (x = y?=w195:bool)
          n143 = Equal?(x="", y=w200) -> (x = y?=w202:bool)
          n144 = Equal?(x="", y=w207) -> (x = y?=w209:bool)
          n145 = Select(t="STOP", s=w174, f=w172) -> (s? t:f=w171:string)
          n146 = Select(t="STOP", s=w181, f=w179) -> (s? t:f=w178:string)
          n147 = Select(t="STOP", s=w188, f=w186) -> (s? t:f=w185:string)
          n148 = Select(t="STOP", s=w195, f=w193) -> (s? t:f=w192:string)
          n149 = Select(t="STOP", s=w202, f=w200) -> (s? t:f=w199:string)
          n150 = Select(t="STOP", s=w209, f=w207) -> (s? t:f=w205:string)
          n151 = Bundle(cluster=w170, "STATUS"=w171) -> (w169:T4)  [unwired: 2 in]
          n152 = Bundle(cluster=w177, "STATUS"=w178) -> (w176:T4)  [unwired: 2 in]
          n153 = Bundle(cluster=w184, "STATUS"=w185) -> (w183:T4)  [unwired: 2 in]
          n154 = Bundle(cluster=w191, "STATUS"=w192) -> (w190:T4)  [unwired: 2 in]
          n155 = Bundle(cluster=w197, "STATUS"=w199) -> (w198:T4)  [unwired: 2 in]
          n156 = Bundle(cluster=w206, "STATUS"=w205) -> (w204:T4)  [unwired: 2 in]
          n157 = local write "DISP LAB01-2"(w198) -> ()
          n158 = local write "DISP LAB01-1"(w204) -> ()
          n159 = local write "DISP LAB02-1"(w190) -> ()
          n160 = local write "DISP LAB03-1"(w176) -> ()
          n161 = local write "DISP LAB02-2"(w183) -> ()
          n162 = local write "DISP LAB03-2"(w169) -> ()
          n163 = local read "DISP LAB05-2"() -> (w142:T4)
          n164 = local read "DISP LAB05-1"() -> (w149:T4)
          n165 = local read "DISP LAB04-2"() -> (w151:T4)
          n166 = local read "DISP LAB04-1"() -> (w153:T4)
          n167 = Unbundle(w142) -> ("STATUS"=w144:string)  [unwired: 2 out]
          n168 = Unbundle(w149) -> ("STATUS"=w155:string)  [unwired: 2 out]
          n169 = Unbundle(w151) -> ("STATUS"=w160:string)  [unwired: 2 out]
          n170 = Unbundle(w153) -> ("STATUS"=w165:string)  [unwired: 2 out]
          n171 = Equal?(x="", y=w144) -> (x = y?=w146:bool)
          n172 = Equal?(x="", y=w155) -> (x = y?=w157:bool)
          n173 = Equal?(x="", y=w160) -> (x = y?=w162:bool)
          n174 = Equal?(x="", y=w165) -> (x = y?=w167:bool)
          n175 = Select(t="STOP", s=w146, f=w144) -> (s? t:f=w143:string)
          n176 = Select(t="STOP", s=w157, f=w155) -> (s? t:f=w154:string)
          n177 = Select(t="STOP", s=w162, f=w160) -> (s? t:f=w159:string)
          n178 = Select(t="STOP", s=w167, f=w165) -> (s? t:f=w164:string)
          n179 = Bundle(cluster=w142, "STATUS"=w143) -> (w141:T4)  [unwired: 2 in]
          n180 = Bundle(cluster=w149, "STATUS"=w154) -> (w148:T4)  [unwired: 2 in]
          n181 = Bundle(cluster=w151, "STATUS"=w159) -> (w150:T4)  [unwired: 2 in]
          n182 = Bundle(cluster=w153, "STATUS"=w164) -> (w152:T4)  [unwired: 2 in]
          n183 = local write "DISP LAB05-2"(w141) -> ()
          n184 = local write "DISP LAB05-1"(w148) -> ()
          n185 = local write "DISP LAB04-1"(w152) -> ()
